vi "Get Config.vi"(8 "error in (no error)":errorcluster, 11 "MSX-E3711 in":refnum<class "MSX-E3711.lvclass">) -> (0 "error out":errorcluster, 1 "Config Data":variant, 3 "MSX-E3711 out":refnum<class "MSX-E3711.lvclass">)   [LabVIEW 2014, in "MSX-E3711.lvlib" / "MSX-E3711.lvclass"]
uses:
  MSX-E3711.lvclass
  MSX-E3711.lvclass/MSX-E3711.ctl
  DriverMasterSync/build/DriverMasterSync.lvlibp/Modules/HAL/DriverMasterSync/DriverMasterSyncClass/DriverMasterSync.lvclass
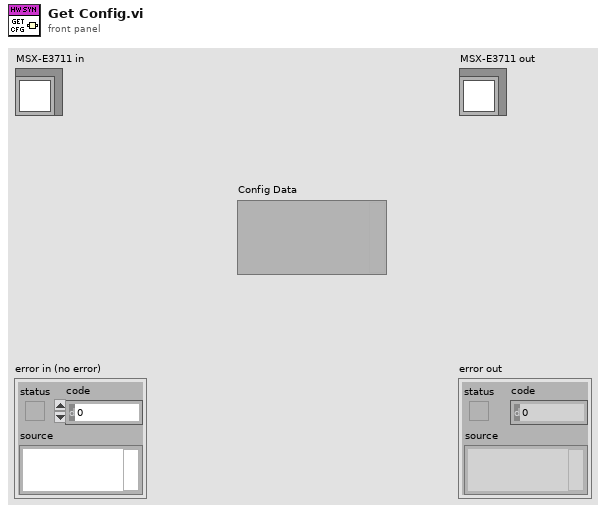
[diagram p1: front panel]
types:
  T1 = typedef "DriverMasterSync.lvlibp/HAL Config Data.ctl" = cluster{"HWSync Index":u32, "Driver Name":string, "Channel Mask":u64}
  T2 = typedef "MSX-E3711_dll.lvlib/Adquisition Data.ctl" = cluster{"Adq. Sequence":cluster{"Adquisition Value":u32[][], "Counter Value":u32[], "TSs - TSu - NAS":u64[][], "Status IO Port":bool[]}, "Adq. Auto Refresh":cluster{"Adquisition Value":u64[], "Status IO Port":bool[], "Counter value":u32}}
  T3 = typedef "MSX-E3711_dll.lvlib/Config Data.ctl" = cluster{"Auto Refresh":cluster{"Average Mode":u64, "Average Value":u64, "Trigger Mask":u64, "Trigger Mode":u64, "Hardware Trigger Edge":u64, "Hardware Trigger Count":u64, "By Trigger Nbr Of Seq To Acquire":u64, "Time stamp":bool, "Analog Output(mm)":bool, "Invert value":bool, "Temperature value":bool, "Incremental counter value":bool, "Diff. mode":bool}, "Gain":sgl[], "Offset":sgl[], "Index":u64, "Range":sgl, "Sequence":cluster{"Nbr Of Sequence":u64, "Nbr Max Sequence To Transfer":u64, "Delay Mode":u64, "Delay Time Unit":u64, "Delay Value":u64, "Trigger Mask":u64, "Trigger Mode":u64, "Hardware Trigger Edge":u64, "Hardware Trigger Count":u64, "By Trigger Nbr Of Seq To Acquire":u64, "Time stamp":bool, "Sequence counter information":bool, "Analog Output(mm)":bool, "Invert value":bool, "Temperature value":bool, "Incremental counter value":bool, "Diff. mode":bool}, "Enable DIO":bool, "IncCounter":cluster{"CounterMode":string, "CounterOptionDIRECT  ":bool, "CounterOptionOthers":bool, "CounterClear ":bool, "Cantidad de Pulsos":sgl, "Reducción":sgl}, "IncTemperature":cluster{"ConnectedTempSensor":string, "ConvertMode":string, "InitGainSelection":string, "FrequencySelection":string, "PowerSaveMode":bool, "GainSelection":string, "RefValue":dbl}}
  T4 = typedef "MSX-E3711_dll.lvlib/Connection Data.ctl" = cluster{"MX371x refnum":refnum<k24>, "IP":string, "Connection ID ":refnum<k5>, "MXCommon refnum":refnum<k24>}
  T5 = typedef "MSX-E3711_dll.lvlib/Diagnostic Data.ctl" = cluster{"Muestras Diag. Cycle":u32, "Tolerancia Cycle":sgl, "Tolerancia":sgl, "Mask Proteccion T":u64, "Promedio Transd":sgl[]}
  T6 = cluster{"Channel Mask":u64, "Adquisition Data":T2, "Config Data":T3, "Connection Data":T4, "Diagnostic Data":T5}
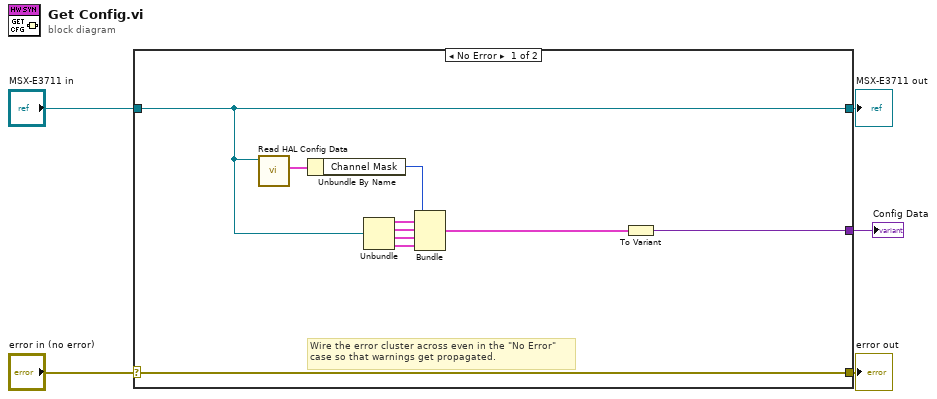
[diagram p0: block diagram]
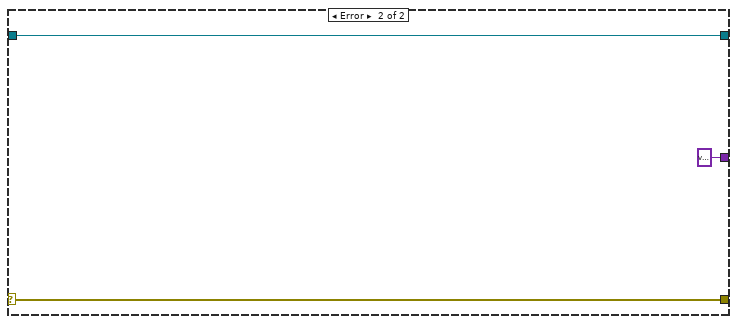
[diagram p2: hidden frame]
diagram:
  n1 = case shown="No Error" "error in (no error)" {
    selector: "error in (no error)" -> [w15 w18]
    tunnel: [w15 w18] -> w4
    tunnel: [w7 w17] -> w2
    tunnel: "MSX-E3711 in" -> [w7 w17]
    tunnel: [w6 variant ("Variant")] -> w1
    frame No Error {
      # "Wire the error cluster across even in the \"No Error\"\ncase so that warnings get propagated."
      n2 = call "Read HAL Config Data.vi"("DriverMasterSync in"=w7) -> ("HAL Config Data"=w8:T1)  [unwired: 8 in, 2 out]
      n3 = Unbundle By Name(w8) -> ("Channel Mask"=w14:u64)
      n4 = Unbundle(w7) -> (w13:T2, w12:T3, w11:T4, w10:T5)
      n5 = Bundle("Channel Mask"=w14, "Adquisition Data"=w13, "Config Data"=w12, "Connection Data"=w11, "Diagnostic Data"=w10) -> (w9:T6)  [unwired: 1 in]
      n6 = To Variant(anything=w9) -> (Variant=w6:variant)
    }
    frame Error {
    }
  }
  "error out" <- w4
  "MSX-E3711 out" <- w2
  "Config Data" <- w1
